vi "RTControl (1).vi"(8 "error in (no error)":errorcluster) -> (0 "error out":errorcluster)   [LabVIEW 2017]
doc: "The \"brain\" of RTMain, where the data is processed and the solenoids are actuated. Contains a finite state machine that determines which stage the pod is in, and emergency check conditions in the event the run must be aborted."
uses:
  StateList.ctl
  <vilib>/Platform/TimedLoop/XDataNode/timing_clust.ctl
  <vilib>/Platform/TimedLoop/XDataNode/nitl_modes.ctl
  <vilib>/Platform/TimedLoop/XDataNode/wakeup.ctl
  SystemToggle/SystemToggleEnum.ctl
  Sensors/DataStreamIndex.ctl
  LoopPeriodGLOBAL.vi
  <vilib>/Platform/TimedLoop/XDataNode/loadnilvce.vi
  ControlTimersGLOBAL.vi
  ForceIdleGLOBAL.vi
  DataTargetsGLOBAL.vi
  ControlActivateSolenoidsGlobal.vi
  StopGLOBAL.vi
  <vilib>/platform/TimedLoop/XDataNode/XDataNode.xnode
  <vilib>/Platform/TimedLoop/XDataNode/XDNodeRunTimeDep.lvlib
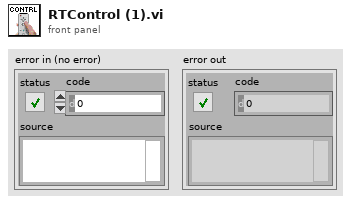
[diagram p1: front panel]
types:
  T1 = typedef "StateList.ctl" = enum16{"Fault", "Idle", "Ready", "Pushing", "Coast", "Braking"}
  T2 = typedef "XDNodeRunTimeDep.lvlib/timing_clust.ctl" = cluster{"Expected End [f-1]":u64, "Actual End [f-1]":u64, "Finished Late? [f-1]":bool, "Expected End [i-1]":u64, "Actual End [i-1]":u64, "Finished Late? [i-1]":bool, "Expected Start [i]":u64, "Actual Start [i]":u64, "Expected Start [f]":u64, "Actual Start [f]":u64, "Source Name":string, "Structure Name":string, "Period":i64, "Deadline":i64, "Offset":i64, "Start":i64, "Priority":i32, "Timeout":i32, "Mode":T3, "Wakeup Reason":T4, "Error":errorcluster, "Source Type":string, "Secondary Source Type":string, "Global End Time":u64, "Global Start Time":u64, "Frame Duration":u64, "Iteration Duration":u64, "Assigned CPU":i32, "I/O Scan Engine Mode":u32}
  T3 = typedef "XDNodeRunTimeDep.lvlib/nitl_modes.ctl" = enum32{"No Change", "Process missed periods, maintain original phase", "Discard missed periods, maintain original phase", "Process missed periods, ignore original phase", "Discard missed periods, ignore original phase"}
  T4 = typedef "XDNodeRunTimeDep.lvlib/wakeup.ctl" = enum32{"Normal", "Aborted", "Asynchronous wakeup", "Timing source error", "Timed loop error", "Timeout"}
  T5 = typedef "SystemToggleEnum.ctl" = enum16{"Idle", "MagBrake", "Suspension", "Levitation", "Run"}
  T6 = typedef "DataStreamIndex.ctl" = enum16{"SuspensionPT (PSI)", "MagBrakePT (PSI)", "Baby HPPT (PSI)", "BigRight HPPT (PSI)", "BigLeft HPPT (PSI)", "HallEffect FrontLeft (V)", "HallEffect FrontRight (V)", "HallEffect BackRight (V)", "HallEffect BackLeft (V)", "LinearPot FrontRight (V)", "LinearPot FrontLeft (V)", "LinearPot BackRight (V)", "LinearPot BackLeft (V)", "Speed (m/s)", "Distance (m)", "Piezo (V)", "Battery Voltage (V)", "Battery Current", "Battery Temperature (C)", "cRIO Temperature (C)", "Right Big Tank Temperature (C)", "Left Big Tank Temperature (C)", "Baby Tank Temperature (C)", "Right Manifold Temperature (C)", "Left Manifold Temperature (C)", "IMU Acceleration (m/s2)", "IMU Pressure (Pa)", "IMU Temperature (C)"}
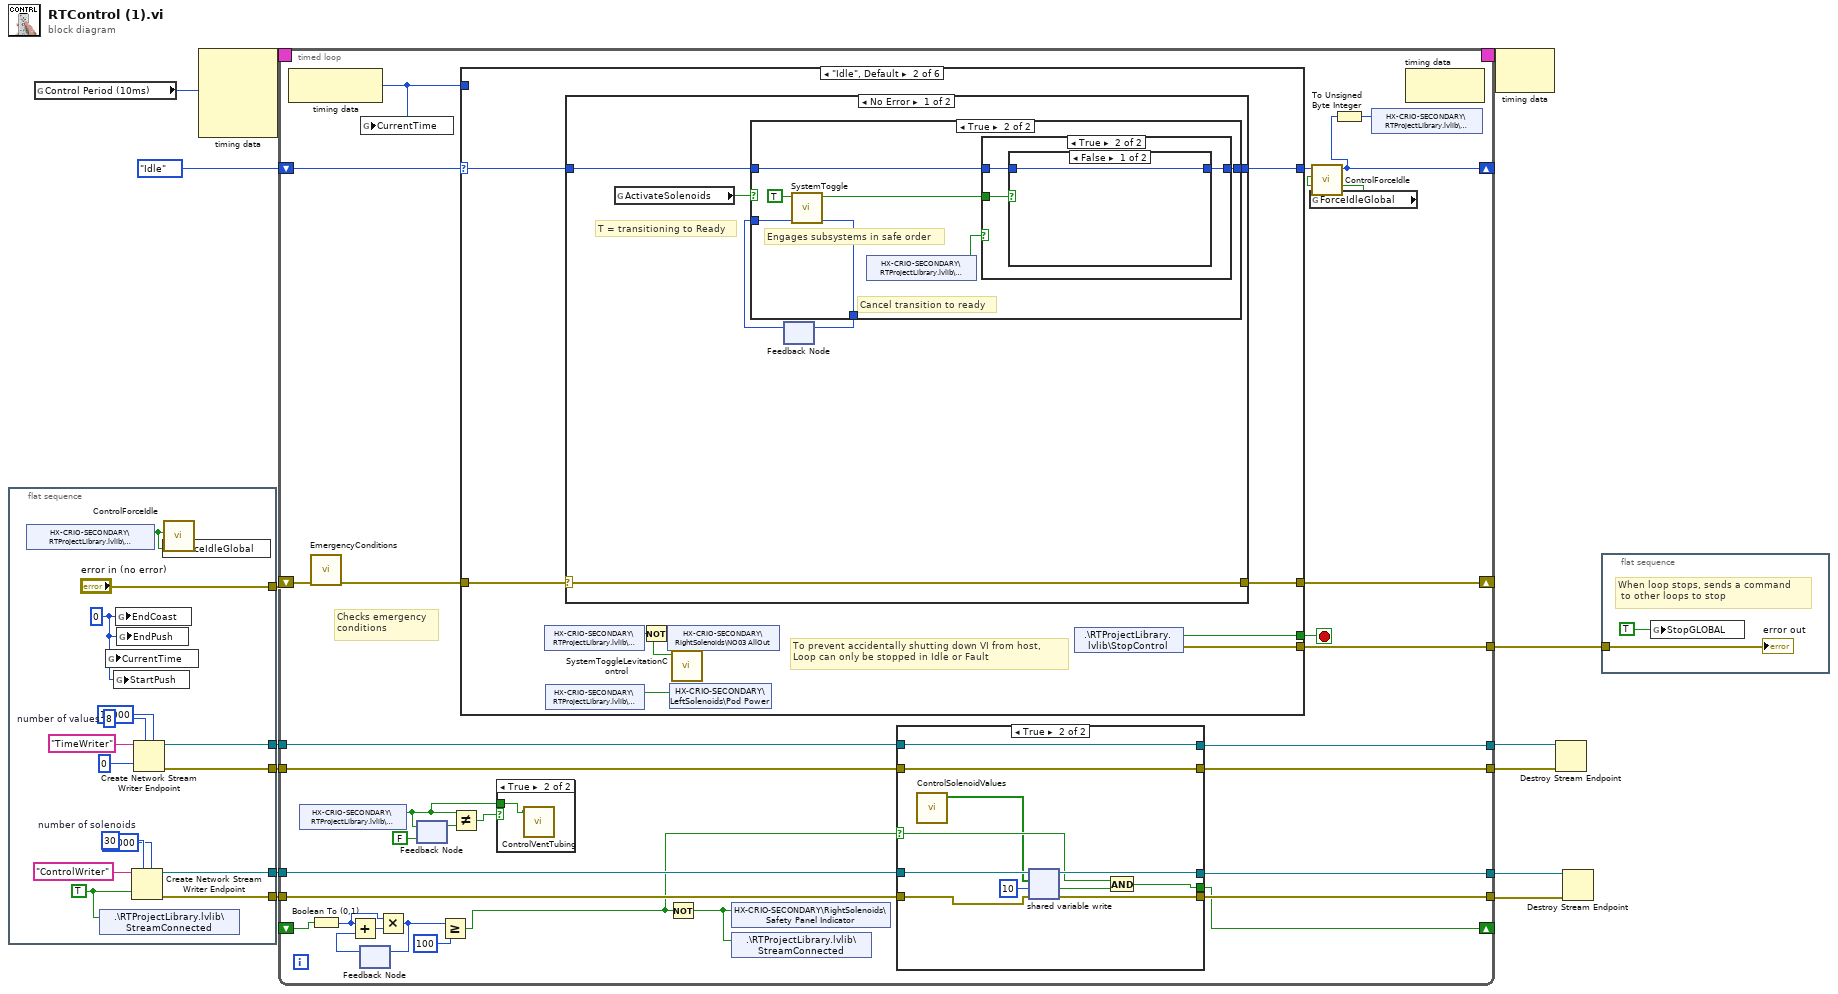
[diagram p0: block diagram]
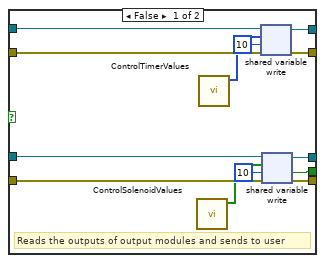
[diagram p2: hidden frame]
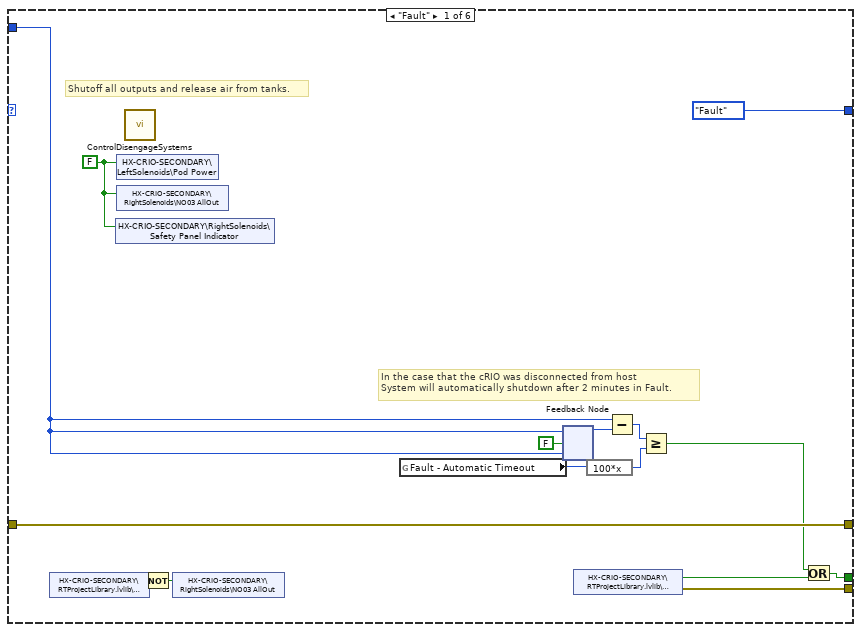
[diagram p4: hidden frame]
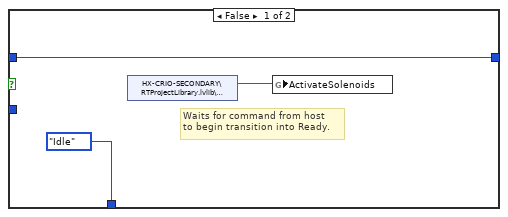
[diagram p5: hidden frame]
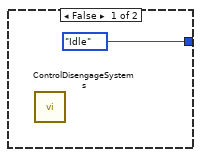
[diagram p6: hidden frame]
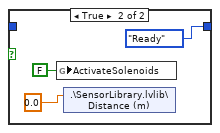
[diagram p7: hidden frame]
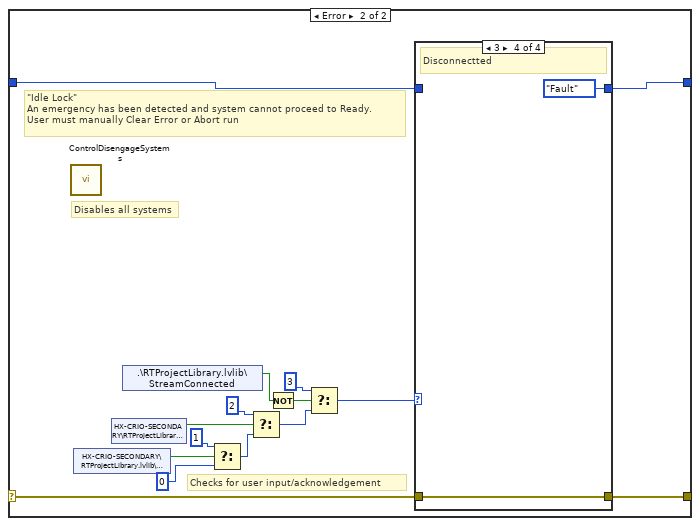
[diagram p8: hidden frame]
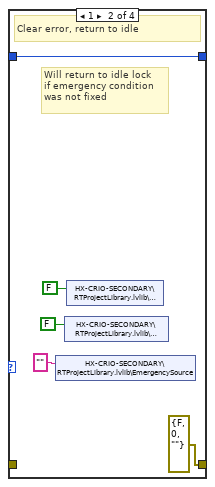
[diagram p10: hidden frame]
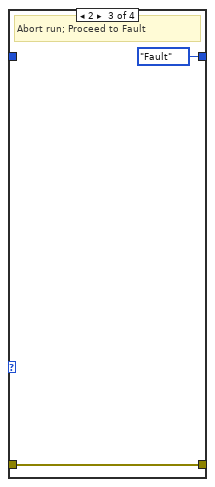
[diagram p11: hidden frame]
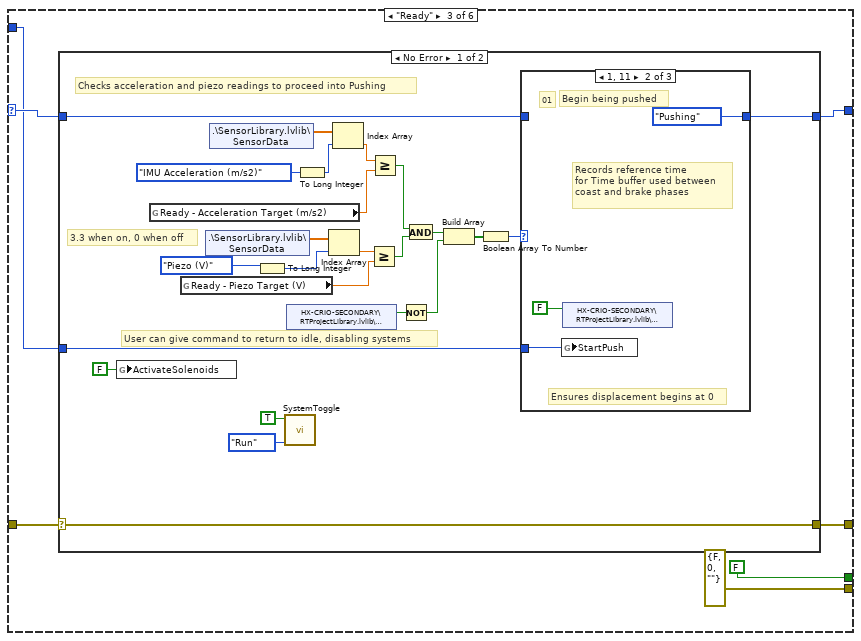
[diagram p12: hidden frame]
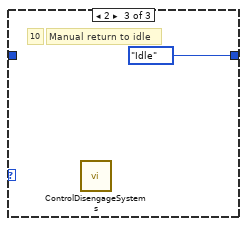
[diagram p14: hidden frame]
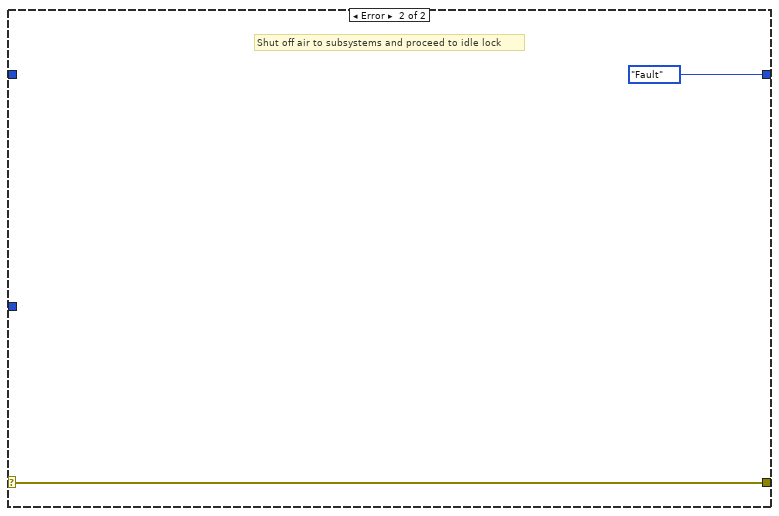
[diagram p15: hidden frame]
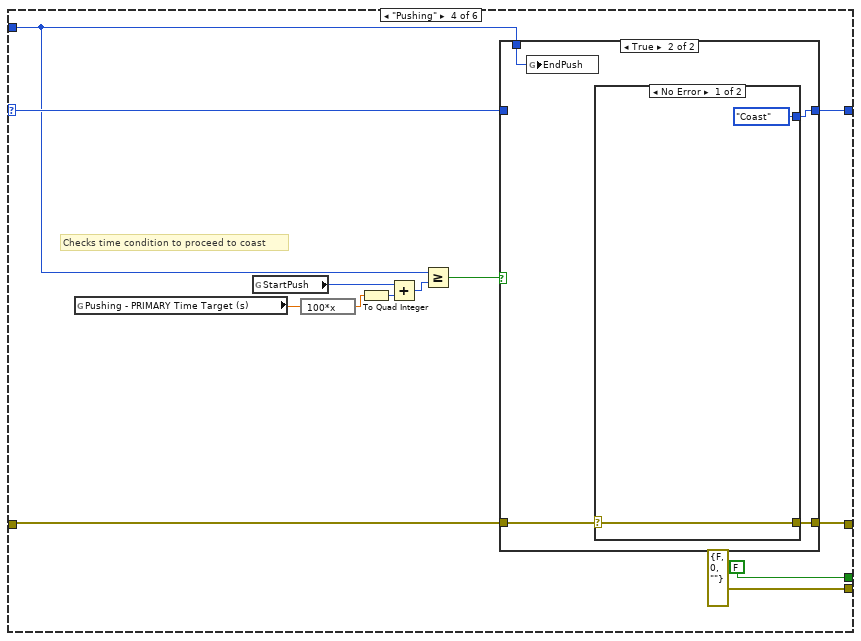
[diagram p16: hidden frame]
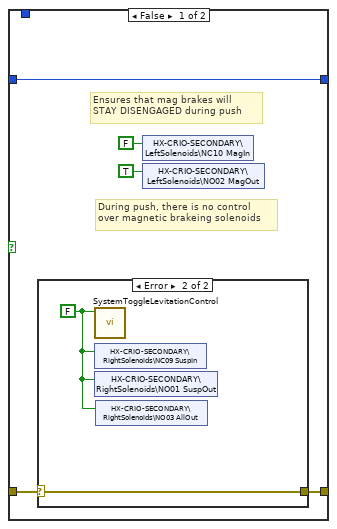
[diagram p17: hidden frame]
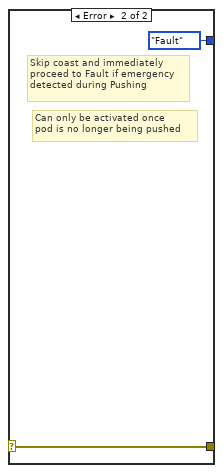
[diagram p19: hidden frame]
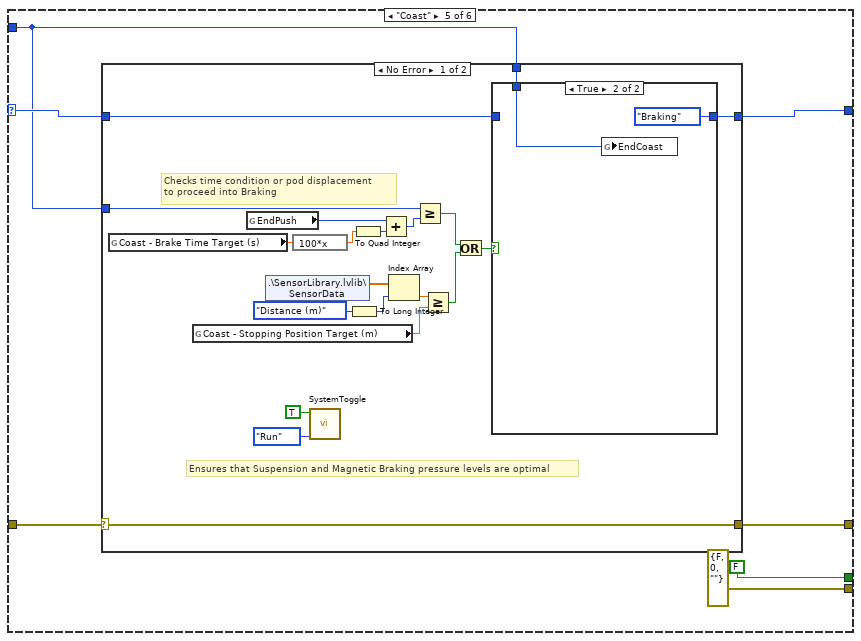
[diagram p20: hidden frame]
diagram:
  n1 = flat-sequence {
    tunnel: [w28] -> w11
    tunnel: [w27] -> w10
    tunnel: ["error in (no error)"] -> w6
    tunnel: [w22] -> w4
    tunnel: [w21] -> w3
    frame #0 {
      w18 = i64 0 ("StartPush")
      w19 = 8  # number of values
      w24 = 30  # number of solenoids
      w20 = TRUE
      n2 = shared-variable "HX-CRIO-SECONDARY\\RTProjectLibrary.lvlib\\EnableForceIdle"() -> (w15:bool)  [unwired: 1 in, 1 out]
      n3 = shared-variable ".\\RTProjectLibrary.lvlib\\StreamConnected"(w20) -> ()  [unwired: 1 in, 1 out]
      n4 = global write "ControlTimersGLOBAL.vi" "CurrentTime"(w18) -> ()
      n5 = global write "ControlTimersGLOBAL.vi" "StartPush"(w18) -> ()
      n6 = global write "ControlTimersGLOBAL.vi" "EndCoast"(w18) -> ()
      n7 = global write "ControlTimersGLOBAL.vi" "EndPush"(w18) -> ()
      n8 = Create Network Stream Writer Endpoint(5:10000 ("timeout in ms (-1)"), 7:w24, 9:w20, 11:"ControlWriter" ("writer name")) -> (0:w27:errorcluster, 3:w28:refnum<k21>)  [unwired: 3 in]
      n9 = Create Network Stream Writer Endpoint(5:10000 ("timeout in ms (-1)"), 7:w19, 9:i64 0, 11:"TimeWriter" ("writer name")) -> (0:w21:errorcluster, 3:w22:refnum<k21>)  [unwired: 3 in]
      n10 = global write "ForceIdleGLOBAL.vi" "ForceIdleGlobal"(w15) -> ()
      n11 = call "ControlForceIdle.vi"("Enabled"=w15) -> ()  [unwired: 10 in, 1 out]
    }
  }
  n12 = global read "LoopPeriodGLOBAL.vi" "Control Period (10ms)"() -> (w5:i64)
  n13 = node-c288(w5) -> (w14:T2)  [unwired: 3 in]
  n14 = timed-loop {
    timing: w14 -> [_]
    timing-out: [_] -> w13
    shift-right: [w45] -> _
    shift-left: StateList."Idle" ("Start Phase") -> [w61]
    tunnel: w11 -> [w52]
    tunnel: w10 -> [w51]
    tunnel: [w60] -> w9
    tunnel: [w59] -> w8
    shift-right: [w58] -> _
    shift-left: w6 -> [w54]
    tunnel: [w55] -> w7
    tunnel: w4 -> [w50]
    tunnel: w3 -> [w30]
    tunnel: [w49] -> w2
    tunnel: [w48] -> w1
    shift-right: [w39] -> _
    shift-left: _ -> [w33]
    stop <- w56 stop-if-true
    # "Checks emergency\nconditions"
    n15 = node-c288() -> (w47:i64)  [unwired: 1 in]
    n16 = shared-variable "HX-CRIO-SECONDARY\\RTProjectLibrary.lvlib\\VentTubing"() -> (w40:bool)  [unwired: 1 in, 1 out]
    n17 = call "EmergencyConditions.vi"("error in (no error)"=w54) -> ("error out"=w53:errorcluster)  [unwired: 10 in]
    n18 = Boolean To (0,1)(Boolean=w33) -> (0, 1=w35:i16)
    n19 = feedback #1() -> (w36:i16)  [unwired: 1 in]
    n20 = Add(x=w35, y=w36) -> (x+y=w34:i16)
    n21 = global write "ControlTimersGLOBAL.vi" "CurrentTime"(w47) -> ()
    n22 = Multiply(x=w35, y=w34) -> (x*y=w37:i16)
    n23 = feedback-in #1(w37) -> ()
    n24 = feedback-in #2(w40) -> ()
    n25 = feedback #2(FALSE ("Boolean")) -> (w43:bool)
    n26 = Greater Or Equal?(x=w37, y=i16 100) -> (x >= y?=w31:bool)
    n27 = Not Equal?(x=w40, y=w43) -> (x != y?=w42:bool)
    n28 = case shown="\"Idle\", Default" w61 {
      selector: w61 -> [_ w110 w167 w211 w234 w266]
      tunnel: w47 -> [w93 _ w166 w199 w228 _]
      tunnel: [StateList."Fault" ("Start Phase") w109 w165 w210 w233 w265] -> w46
      tunnel: w53 -> [w99 w108 w164 w209 w232 w264]
      tunnel: [w99 w107 w163 w208 w231 w263] -> w58
      tunnel: [w98 w106 errorcluster {"status"=FALSE, "code"=0, "source"=""} ("error IO") errorcluster {"status"=FALSE, "code"=0, "source"=""} ("error IO") errorcluster {"status"=FALSE, "code"=0, "source"=""} ("error IO") errorcluster {"status"=FALSE, "code"=0, "source"=""} ("error IO")] -> w55
      tunnel: [w97 w105 FALSE ("Boolean") FALSE ("Boolean") FALSE ("Boolean") FALSE ("Boolean")] -> w56
      frame "Fault" {
        w100 = FALSE ("Pod Power")
        # "In the case that the cRIO was disconnected from host\nSystem will automatically shutdown after 2 minutes in Fault."
        # "Shutoff all outputs and release air from tanks."
        n29 = shared-variable "HX-CRIO-SECONDARY\\RTProjectLibrary.lvlib\\VentTanks"() -> (w88:bool)  [unwired: 1 in, 1 out]
        n30 = shared-variable "HX-CRIO-SECONDARY\\RightSolenoids\\Safety Panel Indicator"(w100) -> ()  [unwired: 1 in, 1 out]
        n31 = shared-variable "HX-CRIO-SECONDARY\\LeftSolenoids\\Pod Power"(w100) -> ()  [unwired: 1 in, 1 out]
        n32 = shared-variable "HX-CRIO-SECONDARY\\RightSolenoids\\NO03 AllOut"(w100) -> ()  [unwired: 1 in, 1 out]
        n33 = call "ControlDisengageSystems.vi"() -> ()  [unwired: 12 in]
        n34 = Not(x=w88) -> (.not. x?=w87:bool)
        n35 = shared-variable "HX-CRIO-SECONDARY\\RightSolenoids\\NO03 AllOut"(w87) -> ()  [unwired: 1 in, 1 out]
        n36 = global read "DataTargetsGLOBAL.vi" "Fault - Automatic Timeout"() -> (w95:i64)
        n37 = feedback-in #3(w93, FALSE) -> ()
        n38 = feedback #3(w93) -> (w94:i64)
        n39 = shared-variable "HX-CRIO-SECONDARY\\RTProjectLibrary.lvlib\\StopControl"() -> (w96:bool, error out=w98:errorcluster)  [unwired: 1 in]
        n40 = expression code="100*x"(w95) -> (w91:i64)
        n41 = Subtract(x=w93, y=w94) -> (x-y=w92:i64)
        n42 = Greater Or Equal?(x=w92, y=w91) -> (x >= y?=w90:bool)
        n43 = Or(x=w90, y=w96) -> (x .or. y?=w97:bool)
      }
      frame "Idle", Default {
        # "To prevent accidentally shutting down VI from host,\nLoop can only be stopped in Idle or Fault"
        n44 = shared-variable "HX-CRIO-SECONDARY\\RTProjectLibrary.lvlib\\VentTanks"() -> (w102:bool)  [unwired: 1 in, 1 out]
        n45 = shared-variable "HX-CRIO-SECONDARY\\RTProjectLibrary.lvlib\\PodPower"() -> (w103:bool)  [unwired: 1 in, 1 out]
        n46 = case shown="No Error" w108 {
          selector: w108 -> [w113 w144]
          tunnel: w110 -> [w116 w141]
          tunnel: [w115 w142] -> w109
          tunnel: [w113 w143] -> w107
          frame No Error {
            # "T = transitioning to Ready"
            n47 = global read "ControlActivateSolenoidsGlobal.vi" "ActivateSolenoids"() -> (w114:bool)
            n48 = feedback #4() -> (w111:T5)  [unwired: 1 in]
            n49 = case shown="True" w114 {
              tunnel: w116 -> [w119 w121]
              tunnel: [w119 w122] -> w115
              tunnel: [SystemToggleEnum."Idle" w124] -> w112
              tunnel: w111 -> [_ w125]
              frame False {
                # "Waits for command from host\nto begin transition into Ready."
                n50 = shared-variable "HX-CRIO-SECONDARY\\RTProjectLibrary.lvlib\\IdleToReady"() -> (w118:bool)  [unwired: 1 in, 1 out]
                n51 = global write "ControlActivateSolenoidsGlobal.vi" "ActivateSolenoids"(w118) -> ()
              }
              frame True {
                # "Cancel transition to ready"
                # "Engages subsystems in safe order"
                n52 = call "SystemToggle.vi"("Enum In"=w125, "Activate/Deactivate System"=TRUE) -> ("Enum Out"=w124:T5, "PrePush Ready"=w120:bool)  [unwired: 8 in]
                n53 = shared-variable "HX-CRIO-SECONDARY\\RTProjectLibrary.lvlib\\IdleToReady"() -> (w123:bool)  [unwired: 1 in, 1 out]
                n54 = case shown="True" w123 {
                  tunnel: w121 -> [_ w130]
                  tunnel: [StateList."Idle" ("Start Phase") w129] -> w122
                  tunnel: w120 -> [_ w128]
                  frame False {
                    n55 = call "ControlDisengageSystems.vi"() -> ()  [unwired: 12 in]
                  }
                  frame True {
                    n56 = case shown="False" w128 {
                      tunnel: [w131 StateList."Ready" ("Start Phase")] -> w129
                      tunnel: w130 -> [w131 _]
                      frame False {
                      }
                      frame True {
                        n57 = global write "ControlActivateSolenoidsGlobal.vi" "ActivateSolenoids"(FALSE ("ActivateSolenoids")) -> ()
                        n58 = shared-variable ".\\SensorLibrary.lvlib\\Distance (m)"(0.0 ("Distance (m)")) -> ()  [unwired: 1 in, 1 out]
                      }
                    }
                  }
                }
              }
            }
            n59 = feedback-in #4(w112) -> ()
          }
          frame Error {
            # "Disables all systems"
            # "Checks for user input/acknowledgement"
            # "\"Idle Lock\"\nAn emergency has been detected and system cannot proceed to Ready.\nUser must manually Clear Error or Abort run"
            n60 = call "ControlDisengageSystems.vi"() -> ()  [unwired: 12 in]
            n61 = shared-variable "HX-CRIO-SECONDARY\\RTProjectLibrary.lvlib\\ClearError"() -> (w149:bool)  [unwired: 1 in, 1 out]
            n62 = shared-variable "HX-CRIO-SECONDARY\\RTProjectLibrary.lvlib\\Abort"() -> (w147:bool)  [unwired: 1 in, 1 out]
            n63 = shared-variable ".\\RTProjectLibrary.lvlib\\StreamConnected"() -> (w136:bool)  [unwired: 1 in, 1 out]
            n64 = Select(t=i8 1, s=w149, f=i8 0) -> (s? t:f=w148:i8)
            n65 = Select(t=i8 2, s=w147, f=w148) -> (s? t:f=w137:i8)
            n66 = Not(x=w136) -> (.not. x?=w135:bool)
            n67 = Select(t=i8 3, s=w135, f=w137) -> (s? t:f=w138:i8)
            n68 = case shown="3" w138 {
              tunnel: w144 -> [w151 _ w158 w159]
              tunnel: [w151 errorcluster {"status"=FALSE, "code"=0, "source"=""} ("error IO") w158 w159] -> w143
              tunnel: [w150 w155 StateList."Fault" ("Start Phase") StateList."Fault" ("Start Phase")] -> w142
              tunnel: w141 -> [w150 w155 _ _]
              frame 0, Default {
                # "Wait in Idle Lock"
              }
              frame 1 {
                # "Will return to idle lock\nif emergency condition\nwas not fixed"
                # "Clear error, return to idle"
                n69 = shared-variable "HX-CRIO-SECONDARY\\RTProjectLibrary.lvlib\\EmergencySource"("" ("EmergencySource")) -> ()  [unwired: 1 in, 1 out]
                n70 = shared-variable "HX-CRIO-SECONDARY\\RTProjectLibrary.lvlib\\Emergency"(FALSE ("Emergency")) -> ()  [unwired: 1 in, 1 out]
                n71 = shared-variable "HX-CRIO-SECONDARY\\RTProjectLibrary.lvlib\\ClearError"(FALSE ("ClearError")) -> ()  [unwired: 1 in, 1 out]
              }
              frame 2 {
                # "Abort run; Proceed to Fault"
              }
              frame 3 {
                # "Disconnectted"
              }
            }
          }
        }
        n72 = Not(x=w102) -> (.not. x?=w104:bool)
        n73 = shared-variable "HX-CRIO-SECONDARY\\RightSolenoids\\NO03 AllOut"(w104) -> ()  [unwired: 1 in, 1 out]
        n74 = shared-variable "HX-CRIO-SECONDARY\\LeftSolenoids\\Pod Power"(w103) -> ()  [unwired: 1 in, 1 out]
        n75 = call "SystemToggleLevitationControl.vi"("LevitationControl"=w102) -> ()  [unwired: 11 in]
        n76 = shared-variable ".\\RTProjectLibrary.lvlib\\StopControl"() -> (w105:bool, error out=w106:errorcluster)  [unwired: 1 in]
      }
      frame "Ready" {
        n77 = case shown="No Error" w164 {
          selector: w164 -> [w177 w197]
          tunnel: w167 -> [w191 _]
          tunnel: w166 -> [w190 _]
          tunnel: [w185 StateList."Fault" ("Phase out")] -> w165
          tunnel: [w177 w197] -> w163
          frame No Error {
            # "User can give command to return to idle, disabling systems"
            # "Checks acceleration and piezo readings to proceed into Pushing"
            # "3.3 when on, 0 when off"
            n78 = global write "ControlActivateSolenoidsGlobal.vi" "ActivateSolenoids"(FALSE ("ActivateSolenoids")) -> ()
            n79 = global read "DataTargetsGLOBAL.vi" "Ready - Acceleration Target (m/s2)"() -> (w174:dbl)
            n80 = global read "DataTargetsGLOBAL.vi" "Ready - Piezo Target (V)"() -> (w173:dbl)
            n81 = shared-variable ".\\SensorLibrary.lvlib\\SensorData"() -> (w189:dbl[])  [unwired: 1 in, 1 out]
            n82 = shared-variable ".\\SensorLibrary.lvlib\\SensorData"() -> (w183:dbl[])  [unwired: 1 in, 1 out]
            n83 = To Long Integer(number=DataStreamIndex."Piezo (V)" ("Data Stream Index")) -> (32bit integer=w176:i32)
            n84 = call "SystemToggle.vi"("Enum In"=SystemToggleEnum."Run", "Activate/Deactivate System"=TRUE) -> ()  [unwired: 8 in, 2 out]
            n85 = shared-variable "HX-CRIO-SECONDARY\\RTProjectLibrary.lvlib\\IdleToReady"() -> (w179:bool)  [unwired: 1 in, 1 out]
            n86 = To Long Integer(number=DataStreamIndex."IMU Acceleration (m/s2)" ("Data Stream Index")) -> (32bit integer=w175:i32)
            n87 = Index Array(array=w189, index=w176) -> (element=w188:dbl)
            n88 = Index Array(array=w183, index=w175) -> (element=w184:dbl)
            n89 = Greater Or Equal?(x=w188, y=w173) -> (x >= y?=w180:bool)
            n90 = Greater Or Equal?(x=w184, y=w174) -> (x >= y?=w181:bool)
            n91 = Not(x=w179) -> (.not. x?=w178:bool)
            n92 = And(x=w181, y=w180) -> (x .and. y?=w182:bool)
            n93 = Build Array(w182, w178) -> (w186:bool[])
            n94 = Boolean Array To Number(Boolean array=w186) -> (number=w187:u32)
            n95 = case shown="1, 11" w187 {
              tunnel: w191 -> [w192 _ _]
              tunnel: [w192 StateList."Pushing" ("Phase out") StateList."Idle" ("Phase out")] -> w185
              tunnel: w190 -> [_ w195 _]
              frame 0, Default {
                # "continue waiting"
              }
              frame 1, 3 {
                # "Ensures displacement begins at 0"
                # "Records reference time\nfor Time buffer used between\ncoast and brake phases"
                # "Begin being pushed"
                # "01"
                n96 = global write "ControlTimersGLOBAL.vi" "StartPush"(w195) -> ()
                n97 = shared-variable "HX-CRIO-SECONDARY\\RTProjectLibrary.lvlib\\IdleToReady"(FALSE ("ActivateSolenoids")) -> ()  [unwired: 1 in, 1 out]
              }
              frame 2 {
                # "Manual return to idle"
                # "10"
                n98 = call "ControlDisengageSystems.vi"() -> ()  [unwired: 12 in]
              }
            }
          }
          frame Error {
            # "Shut off air to subsystems and proceed to idle lock"
          }
        }
      }
      frame "Pushing" {
        # "Checks time condition to proceed to coast"
        n99 = global read "DataTargetsGLOBAL.vi" "Pushing - PRIMARY Time Target (s)"() -> (w201:dbl)
        n100 = global read "ControlTimersGLOBAL.vi" "StartPush"() -> (w205:i64)
        n101 = expression code="100*x"(w201) -> (w204:dbl)
        n102 = To Quad Integer(1:w204) -> (0:w202:i64)
        n103 = Add(x=w205, y=w202) -> (x+y=w203:i64)
        n104 = Greater Or Equal?(x=w199, y=w203) -> (x >= y?=w200:bool)
        n105 = case shown="True" w200 {
          tunnel: w211 -> [w216 _]
          tunnel: [w216 w223] -> w210
          tunnel: w209 -> [w213 w222]
          tunnel: [w212 w221] -> w208
          tunnel: w199 -> [_ w220]
          frame False {
            # "During push, there is no control\nover magnetic brakeing solenoids"
            # "Ensures that mag brakes will \nSTAY DISENGAGED during push"
            n106 = case shown="Error" w213 {
              selector: w213 -> [w217 w219]
              tunnel: [w217 w219] -> w212
              frame No Error {
              }
              frame Error {
                w218 = FALSE ("LevitationControl")
                n107 = call "SystemToggleLevitationControl.vi"("LevitationControl"=w218) -> ()  [unwired: 11 in]
                n108 = shared-variable "HX-CRIO-SECONDARY\\RightSolenoids\\NC09 SuspIn"(w218) -> ()  [unwired: 1 in, 1 out]
                n109 = shared-variable "HX-CRIO-SECONDARY\\RightSolenoids\\NO01 SuspOut"(w218) -> ()  [unwired: 1 in, 1 out]
                n110 = shared-variable "HX-CRIO-SECONDARY\\RightSolenoids\\NO03 AllOut"(w218) -> ()  [unwired: 1 in, 1 out]
              }
            }
            n111 = shared-variable "HX-CRIO-SECONDARY\\LeftSolenoids\\NC10 MagIn"(FALSE ("NC10 MagIn")) -> ()  [unwired: 1 in, 1 out]
            n112 = shared-variable "HX-CRIO-SECONDARY\\LeftSolenoids\\NO02 MagOut"(TRUE ("NO02 MagOut")) -> ()  [unwired: 1 in, 1 out]
          }
          frame True {
            n113 = global write "ControlTimersGLOBAL.vi" "EndPush"(w220) -> ()
            n114 = case shown="No Error" w222 {
              selector: w222 -> [w224 w227]
              tunnel: [StateList."Coast" ("Start Phase") StateList."Fault" ("Start Phase")] -> w223
              tunnel: [w224 w227] -> w221
              frame No Error {
              }
              frame Error {
                # "Can only be activated once\npod is no longer being pushed"
                # "Skip coast and immediately\nproceed to Fault if emergency\ndetected during Pushing"
              }
            }
          }
        }
      }
      frame "Coast" {
        n115 = case shown="No Error" w232 {
          selector: w232 -> [w244 w260]
          tunnel: w228 -> [w254 _]
          tunnel: w234 -> [w246 _]
          tunnel: [w245 StateList."Fault" ("Start Phase")] -> w233
          tunnel: [w244 w260] -> w231
          tunnel: w228 -> [w235 w258]
          frame No Error {
            # "Ensures that Suspension and Magnetic Braking pressure levels are optimal"
            # "Checks time condition or pod displacement\nto proceed into Braking"
            n116 = global read "DataTargetsGLOBAL.vi" "Coast - Brake Time Target (s)"() -> (w239:dbl)
            n117 = global read "DataTargetsGLOBAL.vi" "Coast - Stopping Position Target (m)"() -> (w238:dbl)
            n118 = global read "ControlTimersGLOBAL.vi" "EndPush"() -> (w253:i64)
            n119 = shared-variable ".\\SensorLibrary.lvlib\\SensorData"() -> (w242:dbl[])  [unwired: 1 in, 1 out]
            n120 = expression code="100*x"(w239) -> (w252:dbl)
            n121 = call "SystemToggle.vi"("Enum In"=SystemToggleEnum."Run", "Activate/Deactivate System"=TRUE) -> ()  [unwired: 8 in, 2 out]
            n122 = To Long Integer(number=DataStreamIndex."Distance (m)" ("Data Stream Index")) -> (32bit integer=w241:i32)
            n123 = To Quad Integer(1:w252) -> (0:w250:i64)
            n124 = Add(x=w253, y=w250) -> (x+y=w251:i64)
            n125 = Index Array(array=w242, index=w241) -> (element=w240:dbl)
            n126 = Greater Or Equal?(x=w254, y=w251) -> (x >= y?=w249:bool)
            n127 = Greater Or Equal?(x=w240, y=w238) -> (x >= y?=w248:bool)
            n128 = Or(x=w249, y=w248) -> (x .or. y?=w247:bool)
            n129 = case shown="True" w247 {
              tunnel: w246 -> [w255 _]
              tunnel: [w255 StateList."Braking" ("Start Phase")] -> w245
              tunnel: w235 -> [_ w256]
              frame False {
              }
              frame True {
                n130 = global write "ControlTimersGLOBAL.vi" "EndCoast"(w256) -> ()
              }
            }
          }
          frame Error {
            n131 = global write "ControlTimersGLOBAL.vi" "EndCoast"(w258) -> ()
          }
        }
      }
      frame "Braking" {
        n132 = case shown="No Error" w264 {
          selector: w264 -> [w268 w299]
          tunnel: w266 -> [w293 _]
          tunnel: [w289 StateList."Fault" ("Start Phase")] -> w265
          tunnel: [w267 w299] -> w263
          frame No Error {
            # "Checks that magnetic brakes have been engaged,\nthe reed switch hasn't been updated in x seconds,\nand acceleration is under an acceptable threshold\nto return to idle."
            n133 = call "SystemToggleMagBrakeControl.vi"("MagBrakeOn?"=FALSE) -> ()  [unwired: 10 in, 1 out]
            n134 = shared-variable ".\\SensorLibrary.lvlib\\SensorData"() -> (w285:dbl[])  [unwired: 1 in, 1 out]
            n135 = shared-variable ".\\SensorLibrary.lvlib\\SensorData"() -> (w274:dbl[])  [unwired: 1 in, 1 out]
            n136 = shared-variable ".\\RTProjectLibrary.lvlib\\StreamConnected"() -> (w269:bool)  [unwired: 1 in, 1 out]
            n137 = To Long Integer(number=DataStreamIndex."Distance (m)" ("Data Stream Index")) -> (32bit integer=w284:i32)
            n138 = global read "DataTargetsGLOBAL.vi" "Braking - PSI Target"() -> (w273:dbl)
            n139 = global read "DataTargetsGLOBAL.vi" "Braking - Time Target(s)"() -> (w278:dbl)
            n140 = global read "DataTargetsGLOBAL.vi" "Braking - Acceleration Target (m/s2)"() -> (w279:dbl)
            n141 = Index Array(array=w285, index=w284) -> (element=w280:dbl)
            n142 = To Long Integer(number=DataStreamIndex."MagBrakePT (PSI)" ("Data Stream Index")) -> (32bit integer=w275:i32)
            n143 = feedback-in #5(w280) -> ()
            n144 = feedback #5() -> (w281:dbl)  [unwired: 1 in]
            n145 = shared-variable ".\\SensorLibrary.lvlib\\SensorData"() -> (w286:dbl[])  [unwired: 1 in, 1 out]
            n146 = Index Array(array=w274, index=w275) -> (element=w272:dbl)
            n147 = Not Equal?(x=w280, y=w281) -> (x != y?=w282:bool)
            n148 = case shown="False" w269 {
              tunnel: w268 -> [_ w295]
              tunnel: [errorcluster {"status"=TRUE, "code"=0, "source"=""} ("error IO") w295] -> w267
              frame False {
              }
              frame True {
              }
            }
            n149 = To Long Integer(number=DataStreamIndex."IMU Acceleration (m/s2)" ("Data Stream Index")) -> (32bit integer=w283:i32)
            n150 = call "Elapsed Time2"("Time Target (s)"=w278, "Reset"=w282) -> ("Time has Elapsed"=w290:bool)  [unwired: 10 in, 7 out]
            n151 = Less Or Equal?(x=w272, y=w273) -> (x <= y?=w271:bool)
            n152 = Index Array(array=w286, index=w283) -> (element=w287:dbl)
            n153 = Greater Or Equal?(x=w287, y=w279) -> (x >= y?=w288:bool)
            n154 = Compound Arithmetic op=AND(w271, w290, w288) -> (w291:bool)
            n155 = case shown="True" w291 {
              tunnel: [w296 StateList."Idle" ("Start Phase")] -> w289
              tunnel: w293 -> [w296 _]
              frame False {
              }
              frame True {
                n156 = call "ControlDisengageSystems.vi"() -> ()  [unwired: 12 in]
              }
            }
          }
          frame Error {
          }
        }
      }
    }
    n157 = case shown="True" w42 {
      tunnel: w40 -> [_ w86]
      frame False {
      }
      frame True {
        n158 = call "ControlVentTubing.vi"("Boolean"=w86) -> ()  [unwired: 11 in]
      }
    }
    n159 = Not(x=w31) -> (.not. x?=w32:bool)
    n160 = shared-variable "HX-CRIO-SECONDARY\\RightSolenoids\\Safety Panel Indicator"(w32) -> ()  [unwired: 1 in, 1 out]
    n161 = shared-variable ".\\RTProjectLibrary.lvlib\\StreamConnected"(w32) -> ()  [unwired: 1 in, 1 out]
    n162 = case shown="True" w31 {
      selector: w31 -> [_ w77]
      tunnel: [w74 w79] -> w60
      tunnel: [w73 w80] -> w59
      tunnel: w52 -> [w72 w82]
      tunnel: w51 -> [w71 w81]
      tunnel: w30 -> [w70 w84]
      tunnel: w50 -> [w69 w85]
      tunnel: [w68 w84] -> w49
      tunnel: [w67 w85] -> w48
      tunnel: [w66 w76] -> w39
      frame False {
        # "Reads the outputs of output modules and sends to user"
        n163 = call "ControlSolenoidValues.vi"() -> ("Solenoids Array"=w63:bool[])  [unwired: 11 in]
        n164 = call "ControlTimerValues.vi"() -> ("Array"=w65:i64[])  [unwired: 11 in]
        n165 = shared-variable-write(w69, w70, w65, 10 ("timeout ms (-1)")) -> (w67:refnum<k21>, w68:errorcluster)  [unwired: 1 out]
        n166 = shared-variable-write(w72, w71, w63, 10 ("timeout ms (-1)")) -> (w74:refnum<k21>, w73:errorcluster, w66:bool)
      }
      frame True {
        n167 = call "ControlSolenoidValues.vi"() -> ("Solenoids Array"=w75:bool[])  [unwired: 11 in]
        n168 = shared-variable-write(w82, w81, w75, 10 ("timeout ms (-1)")) -> (w79:refnum<k21>, w80:errorcluster, w78:bool)
        n169 = And(x=w77, y=w78) -> (x .and. y?=w76:bool)
      }
    }
    n170 = global read "ForceIdleGLOBAL.vi" "ForceIdleGlobal"() -> (w44:bool)
    n171 = call "ControlForceIdle.vi"("Enabled"=w44, "Phase in"=w46) -> ("Phase out"=w45:T1)  [unwired: 9 in]
    n172 = To Unsigned Byte Integer(number=w45) -> (unsigned 8bit integer=w57:u8)
    n173 = shared-variable "HX-CRIO-SECONDARY\\RTProjectLibrary.lvlib\\CurrentState"(w57) -> ()  [unwired: 1 in, 1 out]
    n174 = node-c288() -> ()  [unwired: 1 in, 1 out]
  }
  n175 = node-c288(w13) -> ()  [unwired: 1 out]
  n176 = Destroy Stream Endpoint(8:w2, 11:w1) -> ()  [unwired: 1 out]
  n177 = Destroy Stream Endpoint(8:w8, 11:w9) -> ()  [unwired: 1 out]
  n178 = flat-sequence {
    tunnel: w7 -> [w303]
    frame #0 {
      # "When loop stops, sends a command\n to other loops to stop"
      n179 = global write "StopGLOBAL.vi" "StopGLOBAL"(TRUE ("StopControl")) -> ()
      "error out" <- w303
    }
  }
